vi "Gantry_Driver.vi"(0 "VISA resource name":refnum<visa-resource-name>="COM5", 5 "error in (no error)":errorcluster, 7 "Open Serial":bool, 9 "RO(T)":bool, 11 "Driver-Func":u16(ring)=1 items=["Disable Driver", "Enable Driver", "Read Driver Status"], 13 "Close Serial":bool) -> (6 "FH_NOT(T)":bool, 10 "Enabled(T-RO)":bool, 14 "VISA resource name out":refnum<visa-resource-name>="COM5", 19 "error out":errorcluster)   [LabVIEW 2018]
panel:
  out "Response String Array":string[](array[string])=["01 0 OK IDLE WR 0"]
  out "Driver":string="0"
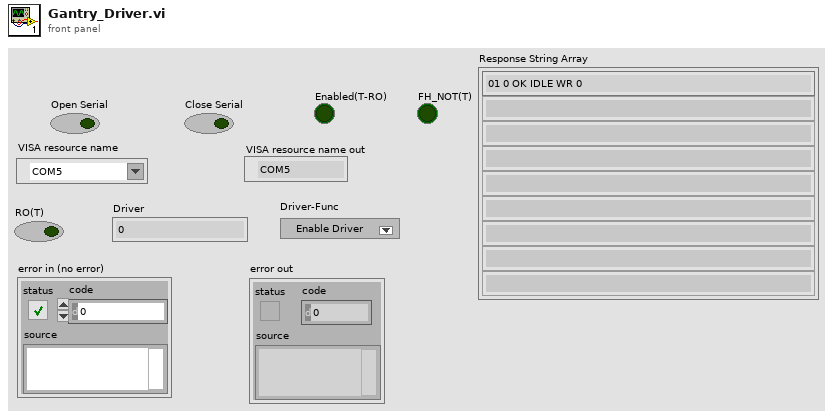
[diagram p1: front panel]
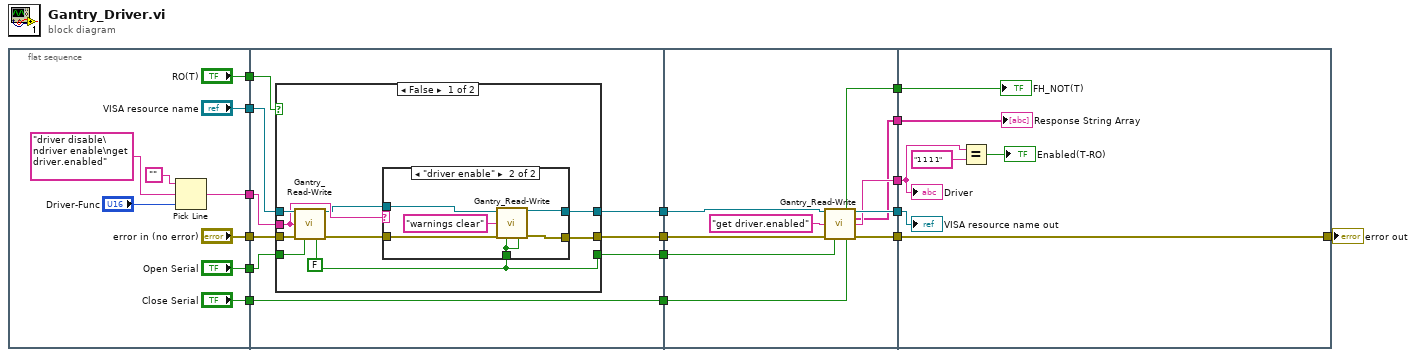
[diagram p0: block diagram]
diagram:
  n1 = flat-sequence {
    tunnel: ["VISA resource name"] -> w16
    tunnel: ["error in (no error)"] -> w15
    tunnel: ["Open Serial"] -> w14
    tunnel: [w22] -> w13
    tunnel: ["Close Serial"] -> w12
    tunnel: ["RO(T)"] -> w4
    tunnel: w16 -> [w34]
    tunnel: w15 -> [w33]
    tunnel: w14 -> [w32]
    tunnel: w13 -> [w31]
    tunnel: w12 -> [w27]
    tunnel: [w30] -> w11
    tunnel: [w29] -> w10
    tunnel: w4 -> [w28]
    tunnel: [w27] -> w2
    tunnel: [w26] -> w1
    tunnel: w11 -> [w63]
    tunnel: w10 -> [w64]
    tunnel: [w59] -> w8
    tunnel: [w58] -> w7
    tunnel: [w57] -> w6
    tunnel: [w62] -> w5
    tunnel: [w61] -> w3
    tunnel: w2 -> [w56]
    tunnel: w1 -> [w55]
    tunnel: [w71] -> w9
    tunnel: w8 -> [w66]
    tunnel: w7 -> [w68]
    tunnel: w6 -> [w69]
    tunnel: w5 -> [w71]
    tunnel: w3 -> [w65]
    frame #0 {
      n2 = Pick Line(string ("")="", multi-line string="driver disable\ndriver enable\nget driver.enabled", line index="Driver-Func") -> (output string=w22:string)
    }
    frame #1 {
      n3 = case shown="False" w28 {
        tunnel: w34 -> [w43 w53]
        tunnel: w33 -> [w42 w54]
        tunnel: w32 -> [w41 w52]
        tunnel: w31 -> [w40 _]
        tunnel: [w37 w54] -> w30
        tunnel: [w36 w53] -> w29
        tunnel: [w35 w52] -> w26
        frame False {
          w35 = FALSE ("Close Serial")
          n4 = call "Gantry_Read-Write.vi"("VISA resource name"=w43, "Command"=w40, "error in (no error)"=w42, "Open Serial"=w41, "Close Serial"=w35) -> ("VISA resource name out"=w39:refnum<visa-resource-name>, "error out"=w38:errorcluster)  [unwired: 4 in, 5 out]
          n5 = case shown="\"driver enable\"" w40 {
            tunnel: w39 -> [w44 w51]
            tunnel: w38 -> [w45 w50]
            tunnel: [w45 w49] -> w37
            tunnel: [w44 w48] -> w36
            tunnel: w35 -> [_ w46]
            frame "False", Default {
            }
            frame "driver enable" {
              n6 = call "Gantry_Read-Write.vi"("VISA resource name"=w51, "Command"="warnings clear", "error in (no error)"=w50, "Open Serial"=w46, "Close Serial"=w46) -> ("VISA resource name out"=w48:refnum<visa-resource-name>, "error out"=w49:errorcluster)  [unwired: 4 in, 5 out]
            }
          }
        }
        frame True {
        }
      }
    }
    frame #2 {
      n7 = call "Gantry_Read-Write.vi"("VISA resource name"=w64, "Command"="get driver.enabled", "error in (no error)"=w63, "Open Serial"=w55, "Close Serial"=w56) -> ("FH_NOT(T)"=w58:bool, "VISA resource name out"=w61:refnum<visa-resource-name>, "Response String Array"=w57:string[], "Data"=w59:string, "error out"=w62:errorcluster)  [unwired: 4 in, 2 out]
    }
    frame #3 {
      n8 = Equal?(x=w66, y="1 1 1 1") -> (x = y?=→"Enabled(T-RO)":bool)
      "Driver" <- w66
      "VISA resource name out" <- w65
      "FH_NOT(T)" <- w68
      "Response String Array" <- w69
    }
  }
  "error out" <- w9
